vi "CRC Verification.vi"(11 "Array":u16[](array[numeric])) -> (0 "CRCL":u8, 1 "CRCH":u8, 2 "CRCL_Rx":u16, 3 "CRCH_Rx":u16, 4 "CRC count":u8)   [LabVIEW 2020]
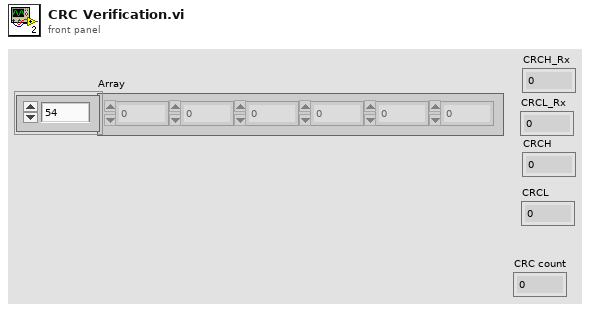
[diagram p1: front panel]
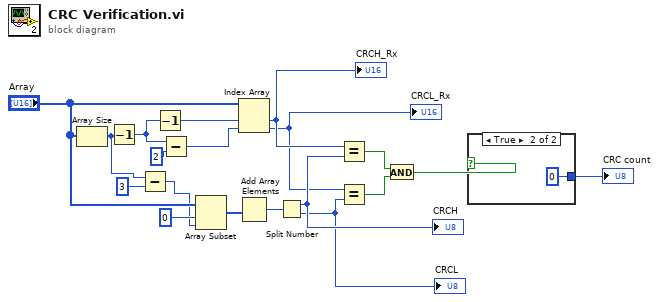
[diagram p0: block diagram]
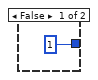
[diagram p2: hidden frame]
diagram:
  n1 = Array Size(array="Array") -> (size(s)=w12:i32)
  n2 = Decrement(x=w12) -> (x-1=w16:i32)
  n3 = Subtract(x=w12, y=3) -> (x-y=w11:i32)
  n4 = Decrement(x=w16) -> (x-1=w19:i32)
  n5 = Subtract(x=w16, y=2) -> (x-y=w17:i32)
  n6 = Array Subset(array="Array", index=0, length=w11) -> (w10:u16[])
  n7 = Index Array(array="Array", index #1=w19, index #2=w17) -> (element #1=w7:u16, element #2=w5:u16)
  "CRCH_Rx" <- w7
  "CRCL_Rx" <- w5
  n8 = Add Array Elements(numeric array=w10) -> (sum=w9:u16)
  n9 = Split Number(x=w9) -> (hi(x)=w8:u8, lo(x)=w6:u8)
  "CRCH" <- w8
  "CRCL" <- w6
  n10 = Equal?(x=w7, y=w8) -> (x = y?=w4:bool)
  n11 = Equal?(x=w5, y=w6) -> (x = y?=w3:bool)
  n12 = And(x=w4, y=w3) -> (x .and. y?=w2:bool)
  n13 = case shown="True" w2 {
    tunnel: [u8 1 u8 0] -> w1
    frame False {
    }
    frame True {
    }
  }
  "CRC count" <- w1
